vi "report.vi"() -> ()   [LabVIEW 2017]
uses:
  <vilib>/addons/database/Connection.llb/DB Tools Open Connec (Path).vi
  <vilib>/Utility/file.llb/Write Delimited Spreadsheet (string).vi
  <vilib>/addons/database/NI_Database_API.lvlib
panel:
  in  "delete":bool
  in  "Scan Barcode":bool
  out "error out":errorcluster
  in  "error in (no error)":errorcluster
  in  "FROM":timestamp format="%<%x>T"
  in  "TO":timestamp format="%<%x>T"
  out "table":string[][](table)
  out "Table header":string[](array[string])
  in  "Barcode":string
  in  "Type Wise":enum16{"Barcode Wise", "Datewise"}(ring)=enum."Datewise"
  in  "stop":bool
  in  "Export to Excel":bool
  in  "Get Report":bool
  # "Data History"
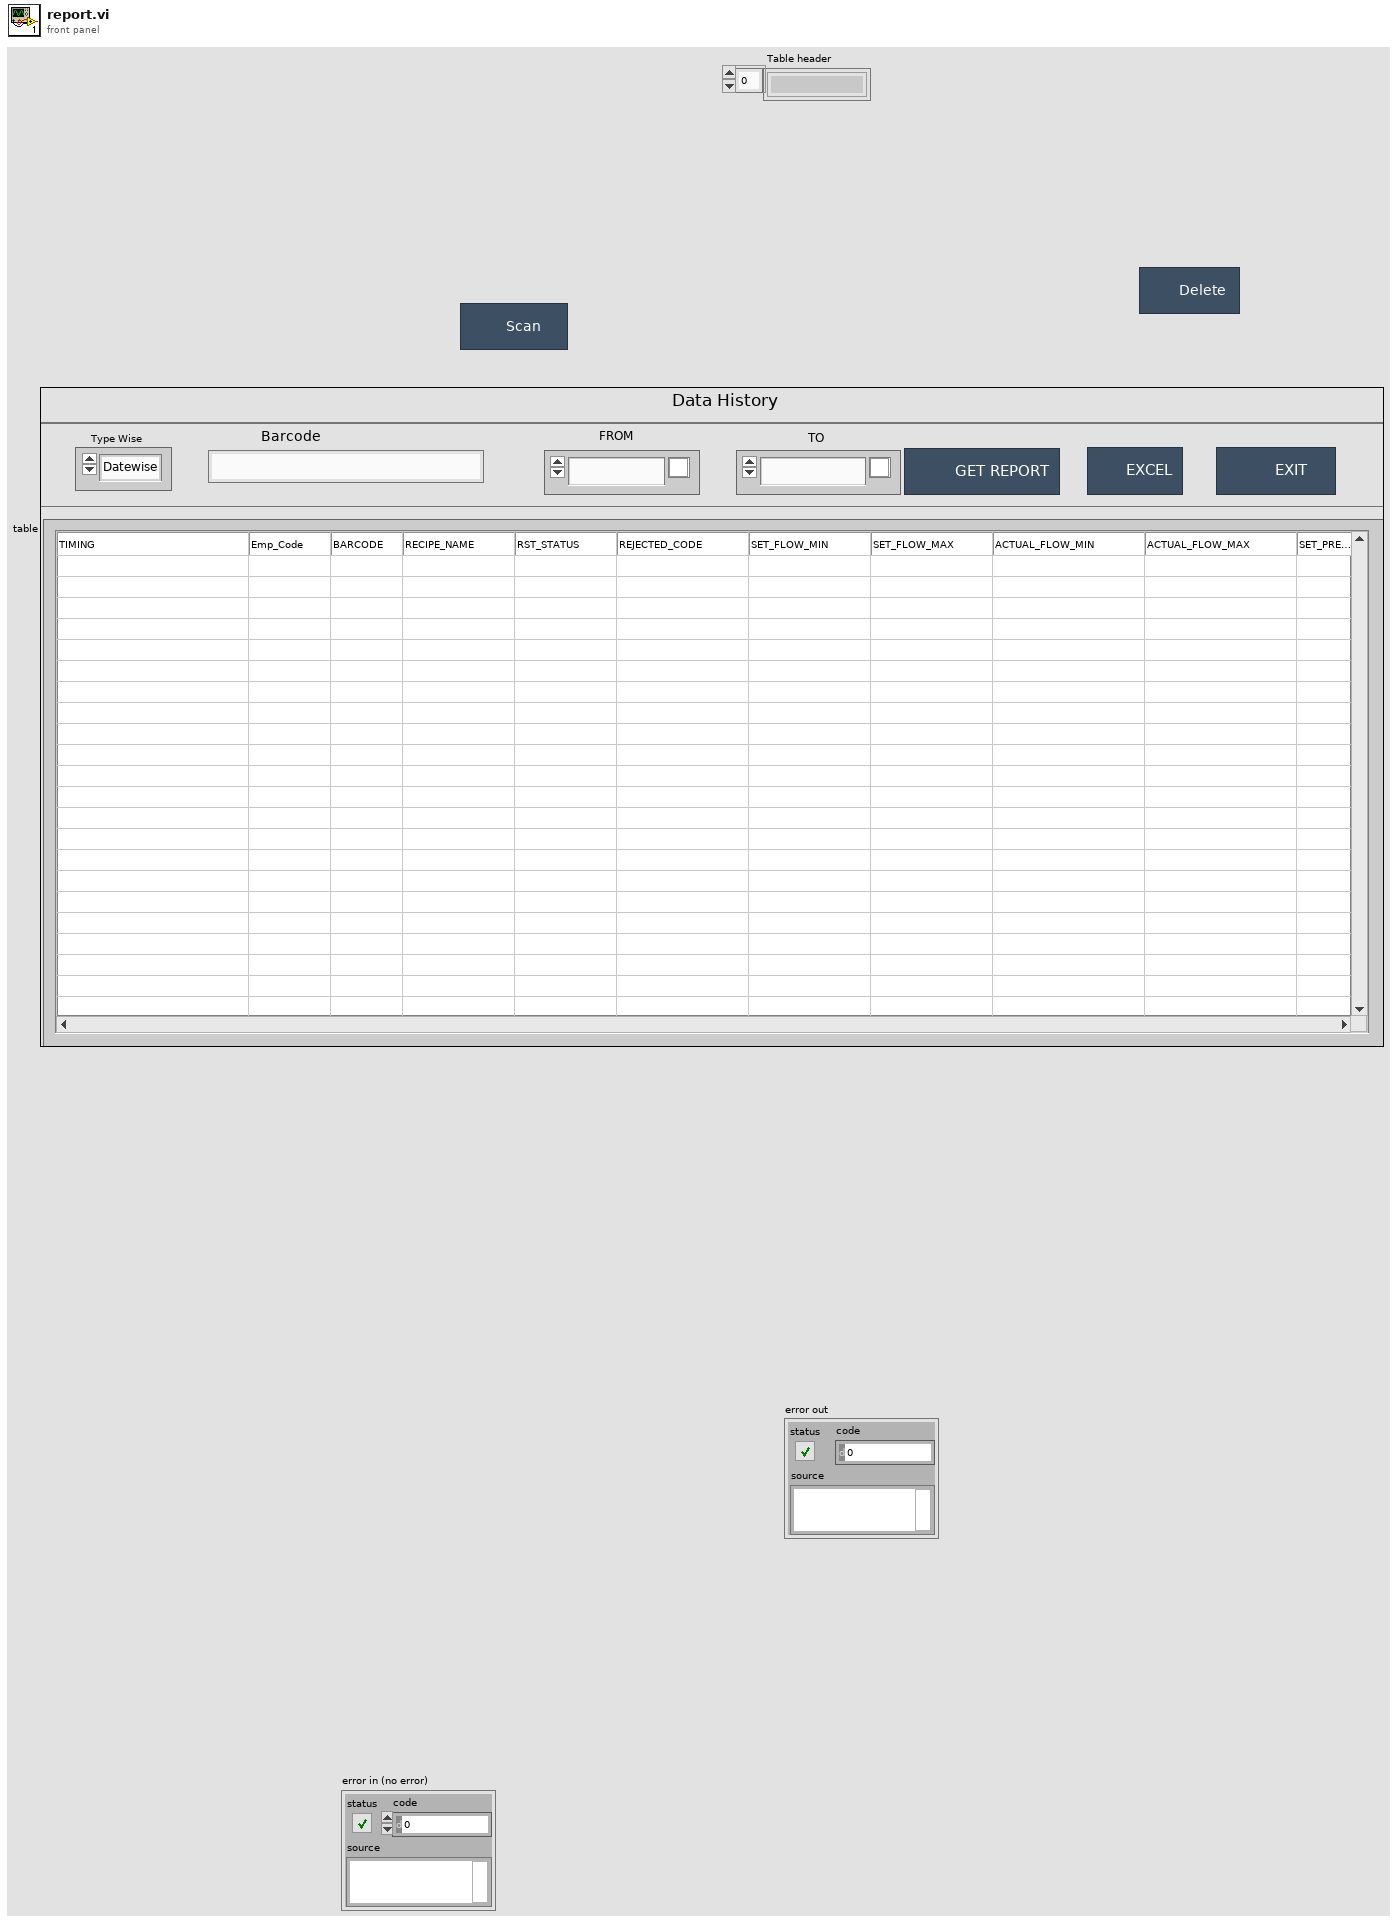
[diagram p1: front panel]
types:
  T1 = typedef "LVDateTimeRec.ctl" = cluster{"fractional second":dbl, "second":i32, "minute":i32, "hour":i32, "day of month":i32, "month":i32, "year":i32, "day of week":i32, "day of year":i32, "DST":i32}
  T2 = typedef "NI_Database_API.lvlib/Conn ObjectReference.ctl" = refnum<k1>
  T3 = enum32{"invalid app kind", "Development System", "Run Time System", "Student Edition", "Embedded LabVIEW", "Evaluation", "Custom"}
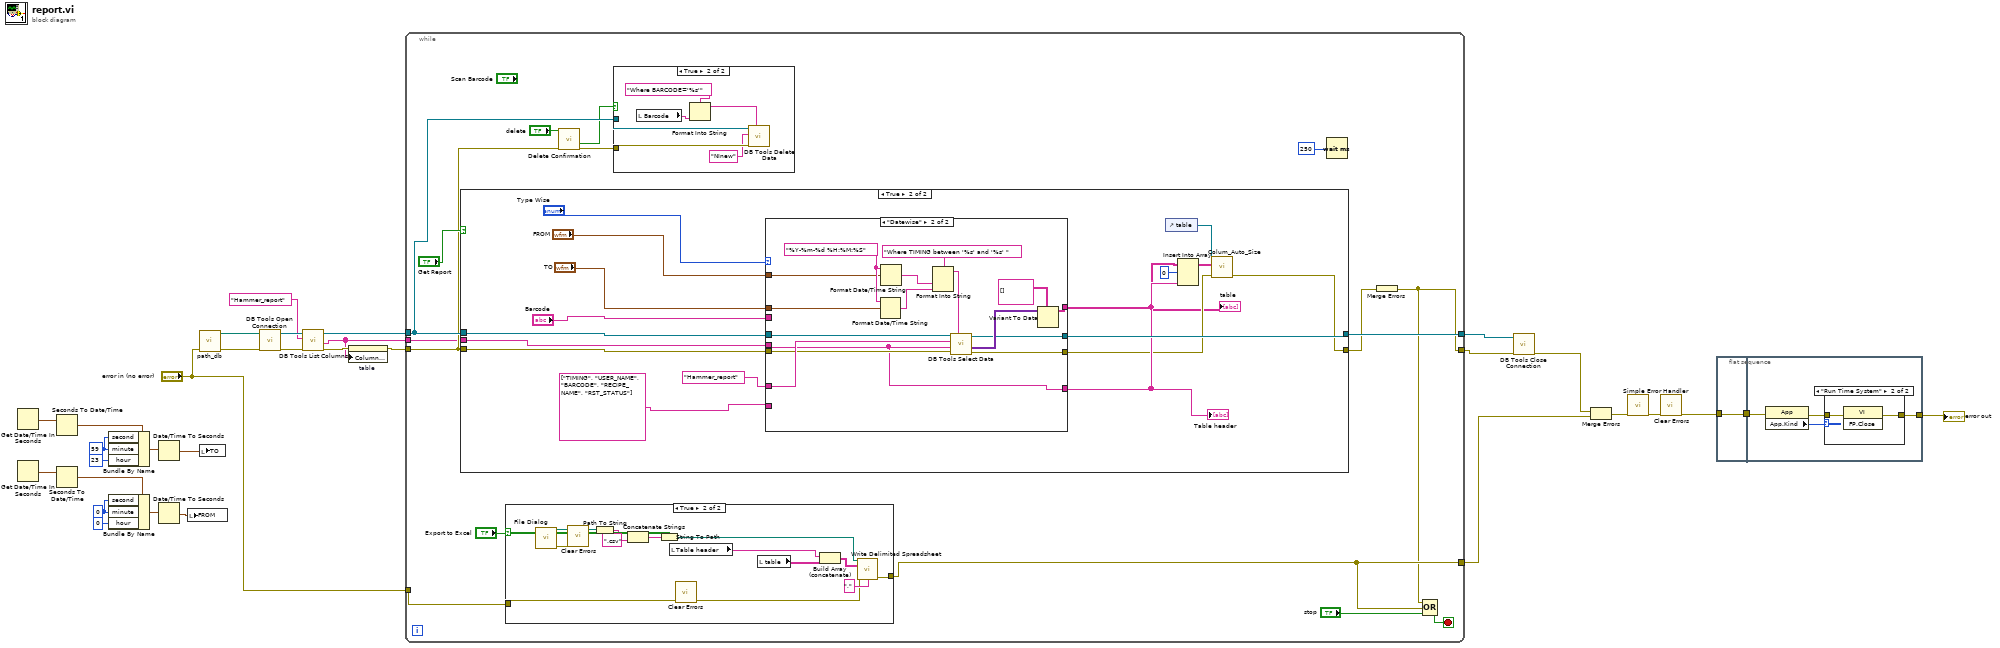
[diagram p0: block diagram]
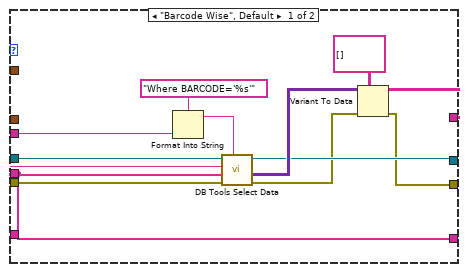
[diagram p6: hidden frame]
diagram:
  w25 = 0 ("minute")
  w26 = 59 ("minute")
  n1 = Get Date/Time In Seconds() -> (seconds since 1Jan1904=w28:timestamp)
  n2 = Get Date/Time In Seconds() -> (seconds since 1Jan1904=w23:timestamp)
  n3 = Seconds To Date/Time(time stamp (now)=w28) -> (date time rec=w29:T1)  [unwired: 1 in]
  n4 = Seconds To Date/Time(time stamp (now)=w23) -> (date time rec=w22:T1)  [unwired: 1 in]
  n5 = Bundle By Name(cluster=w29, "second"=w26, "minute"=w26, "hour"=23) -> (w30:T1)
  n6 = Bundle By Name(cluster=w22, "second"=w25, "minute"=w25, "hour"=0) -> (w21:T1)
  n7 = Date/Time To Seconds(2:w30) -> (0:w19:timestamp)  [unwired: 1 in]
  n8 = Date/Time To Seconds(2:w21) -> (0:w20:timestamp)  [unwired: 1 in]
  n9 = local write "FROM"(w20) -> ()
  n10 = call "path_db.vi"("error in"="error in (no error)") -> ("error out"=w13:errorcluster, "resulting string"=w14:path)  [unwired: 9 in]
  n11 = local write "TO"(w19) -> ()
  n12 = call-poly <vilib>:"DB Tools Open Connection.vi"("error in (no error)"=w13, "connection information"=w14) -> ("error out"=w10:errorcluster, "connection reference"=w9:T2)  [unwired: 6 in]
  n13 = call <vilib>:"DB Tools List Columns.vi"("error in (no error)"=w10, "table"="Hammer_report", "connection reference"=w9) -> ("error out"=w6:errorcluster, "columns"=w4:string[], "connection reference out"=w8:T2)  [unwired: 1 in, 1 out]
  n14 = property on="table" class="Tbl (strict)"(error in=w6, "Column Headers[]"=w4) -> (error out=w5:errorcluster)  [unwired: 1 in, 1 out]
  n15 = while {
    tunnel: w8 -> [w42]
    tunnel: w5 -> [w41]
    tunnel: [w47] -> w18
    tunnel: [w33] -> w11
    tunnel: "error in (no error)" -> [w46]
    tunnel: [w35] -> w16
    tunnel: w4 -> [w37]
    stop <- w32 stop-if-true
    n16 = case shown="True" "Get Report" {
      tunnel: w42 -> [w69 w85]
      tunnel: w41 -> [w68 w84]
      tunnel: [w69 w83] -> w47
      tunnel: [w68 w77] -> w34
      tunnel: w37 -> [_ w70]
      frame False {
      }
      frame True {
        n17 = case shown="\"Datewise\"" "Type Wise" {
          tunnel: w85 -> [w99 w115]
          tunnel: w84 -> [w98 w101]
          tunnel: string[] ["TIMING", "USER_NAME", "BARCODE", "RECIPE_NAME", "RST_STATUS"] -> [_ _]
          tunnel: "Hammer_report" ("table") -> [w93 w112]
          tunnel: [w92 w111] -> w83
          tunnel: [w90 w110] -> w73
          tunnel: [w89 w104] -> w71
          tunnel: [w87 w100] -> w79
          tunnel: "Barcode" -> [w88 _]
          tunnel: "FROM" -> [_ w103]
          tunnel: "TO" -> [_ w102]
          tunnel: w70 -> [w87 w100]
          frame "Barcode Wise", Default {
            n18 = Format Into String(format string="Where BARCODE='%s'", w88) -> (resulting string=w96:string)  [unwired: 2 in, 1 out]
            n19 = call <vilib>:"DB Tools Select Data.vi"("condition"=w96, "error in (no error)"=w98, "columns"=w87, "table"=w93, "connection reference"=w99) -> ("error out"=w91:errorcluster, "data"=w95:variant[][], "connection reference out"=w92:T2)  [unwired: 1 in]
            n20 = Variant To Data(error in=w91, type=string[][] [], Variant=w95) -> (data=w89:string[][], error out=w90:errorcluster)
          }
          frame "Datewise" {
            w106 = "%Y-%m-%d %H:%M:%S" ("time format string (%c)")
            n21 = Format Date/Time String(time format string (%c)=w106, seconds (now)=w102) -> (date/time string=w107:string)  [unwired: 1 in]
            n22 = Format Date/Time String(time format string (%c)=w106, seconds (now)=w103) -> (date/time string=w108:string)  [unwired: 1 in]
            n23 = Format Into String(format string="Where TIMING between '%s' and '%s' ", w108, w107) -> (resulting string=w109:string)  [unwired: 2 in, 1 out]
            n24 = call <vilib>:"DB Tools Select Data.vi"("condition"=w109, "error in (no error)"=w101, "columns"=w100, "table"=w112, "connection reference"=w115) -> ("error out"=w110:errorcluster, "data"=w114:variant[][], "connection reference out"=w111:T2)  [unwired: 1 in]
            n25 = Variant To Data(type=string[][] [], Variant=w114) -> (data=w104:string[][])  [unwired: 1 in, 1 out]
          }
        }
        "table" <- w71
        "Table header" <- w79
        n26 = control-ref of="table"() -> (w76:refnum<vi>)
        n27 = Insert Into Array(array=w71, index (row)=0, new element=w79) -> (w75:string[][])  [unwired: 1 in]
        n28 = call "Colum_Auto_Size.vi"("error in (no error)"=w73, "Table With header"=w75, "Table reference"=w76) -> ("error out"=w77:errorcluster)  [unwired: 8 in]
      }
    }
    n29 = case shown="True" "Export to Excel" {
      tunnel: w46 -> [w54 w67]
      tunnel: [w54 w66] -> w35
      frame False {
      }
      frame True {
        n30 = call "File Dialog"() -> ("selected path"=w60:path, "error out"=w61:errorcluster)  [unwired: 12 in, 2 out]
        n31 = call <vilib>:"Clear Errors.vi"("error in (no error)"=w61) -> ()  [unwired: 5 in, 2 out]
        n32 = Path To String(path=w60) -> (string=w59:string)
        n33 = Concatenate Strings(w59, ".csv" ("string")) -> (w57:string)
        n34 = String To Path(string=w57) -> (path=w56:path)
        n35 = local read "Table header"() -> (w63:string[])
        n36 = call <vilib>:"Clear Errors.vi"("error in (no error)"=w67) -> ("error out"=w55:errorcluster)  [unwired: 5 in, 1 out]
        n37 = local read "table"() -> (w64:string[][])
        n38 = Build Array (concatenate)(w63, w64) -> (w65:string[][])
        n39 = call-poly <vilib>:"Write Delimited Spreadsheet.vi"("file path (dialog if empty)"=w56, "2D data"=w65, "error in (no error)"=w55, "delimiter (\\t)"="," ("delimiter (\\t)")) -> ("error out"=w66:errorcluster)  [unwired: 10 in, 1 out]
      }
    }
    n40 = call "Delete Confirmation"("Enable"="delete", "error in (no error)"=w41) -> ("OK"=w38:bool, "error out"=w40:errorcluster)  [unwired: 16 in]
    n41 = case shown="True" w38 {
      tunnel: w42 -> [_ w53]
      tunnel: w40 -> [_ w52]
      frame False {
      }
      frame True {
        n42 = local read "Barcode"() -> (w51:string)
        n43 = Format Into String(format string="Where BARCODE='%s'", w51) -> (resulting string=w50:string)  [unwired: 2 in, 1 out]
        n44 = call <vilib>:"DB Tools Delete Data.vi"("condition"=w50, "error in (no error)"=w52, "table"="NInew", "connection reference"=w53) -> ()  [unwired: 6 in, 2 out]
      }
    }
    n45 = Wait (ms)(milliseconds to wait=u32 250) -> ()  [unwired: 1 out]
    n46 = Merge Errors(w34) -> (w33:errorcluster)
    n47 = Compound Arithmetic op=OR(w33, w35, "stop") -> (w32:bool)
  }
  n48 = call <vilib>:"DB Tools Close Connection.vi"("error in (no error)"=w11, "connection reference"=w18) -> ("error out"=w17:errorcluster)  [unwired: 5 in]
  n49 = Merge Errors(w17, w16) -> (w3:errorcluster)
  n50 = call <vilib>:"Simple Error Handler.vi"("error in (no error)"=w3) -> ("error out"=w2:errorcluster)  [unwired: 4 in, 4 out]
  n51 = call <vilib>:"Clear Errors.vi"("error in (no error)"=w2) -> ("error out"=w1:errorcluster)  [unwired: 5 in, 1 out]
  n52 = flat-sequence {
    tunnel: w1 -> [w116]
    tunnel: [w116] -> w31
    tunnel: w31 -> [w118]
    tunnel: [w117] -> w15
    frame #0 {
    }
    frame #1 {
      n53 = property class="App"(error in=w118) -> (error out=w119:errorcluster, "App.Kind"=w120:T3)  [unwired: 1 in, 1 out]
      n54 = case shown="\"Run Time System\"" w120 {
        tunnel: w119 -> [w121 w123]
        tunnel: [w121 w122] -> w117
        frame Default {
        }
        frame "Run Time System" {
          n55 = invoke class="VI" method="FP.Close"(error in=w123) -> (error out=w122:errorcluster)  [unwired: 2 in, 2 out]
        }
      }
    }
  }
  "error out" <- w15
